vi "Operaciones.vi"(1 "Operando 2":dbl, 2 "Enum":T1(ring), 3 "Operando 1":dbl) -> (0 "Numeric":dbl)   [LabVIEW 2019]
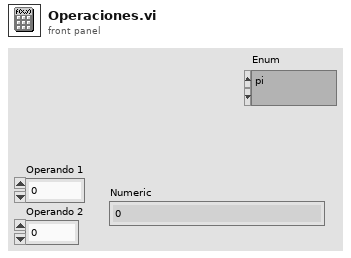
[diagram p1: front panel]
types:
  T1 = enum16{"pi", "Tan^(-1)", "Cos^(-1)", "Sin^(-1)", "Tanh", "Cosh", "Sinh", "Tan", "Cos", "Sin", "x^-1", "x!", "e^x", "Log10", "x^1/k", "x^1/3", "x^1/2", "x^3", "x^2", "Log_x", "x^y", "e", "ln", "/", "x", "+", "-"}
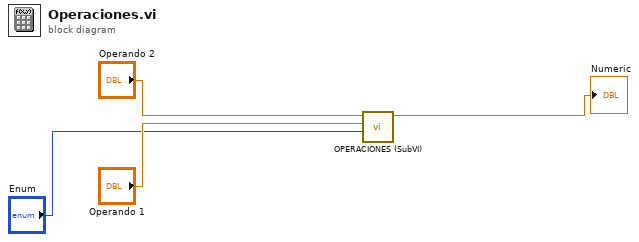
[diagram p0: block diagram]
diagram:
  n1 = call "OPERACIONES (SubVI).vi"("Enum"="Enum", "Operando 1"="Operando 1", "Operando in"="Operando 2") -> ("n!"=→"Numeric":dbl)  [unwired: 8 in]
